vi "Controller Board Thermal Test.vi"(9 "Line In Voltage":dbl format="%#_13g", 10 "Power Supply In":string, 11 "DMM In":string) -> (3 "Temperature":dbl)   [LabVIEW 2013]
doc: "After applying maximum voltage and maximum ambient temperature, measure the temperature of the controller board."
uses:
  <instrlib>/Driver Simulation/DMM/TemperatureSensorTypes.ctl
  <instrlib>/Driver Simulation/Fixture.lvlib
  <instrlib>/Driver Simulation/Power Supply.lvlib
  <instrlib>/Driver Simulation/DMM.lvlib
panel:
  out "error out":errorcluster
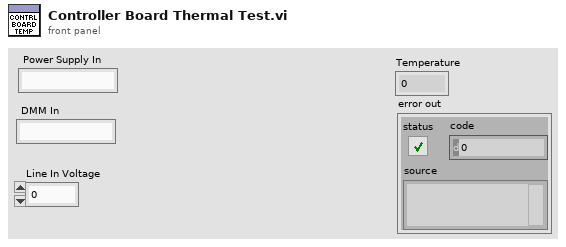
[diagram p1: front panel]
types:
  T1 = typedef "Driver Simulation.lvlib/DMM.lvlib/TemperatureSensorTypes.ctl" = i32
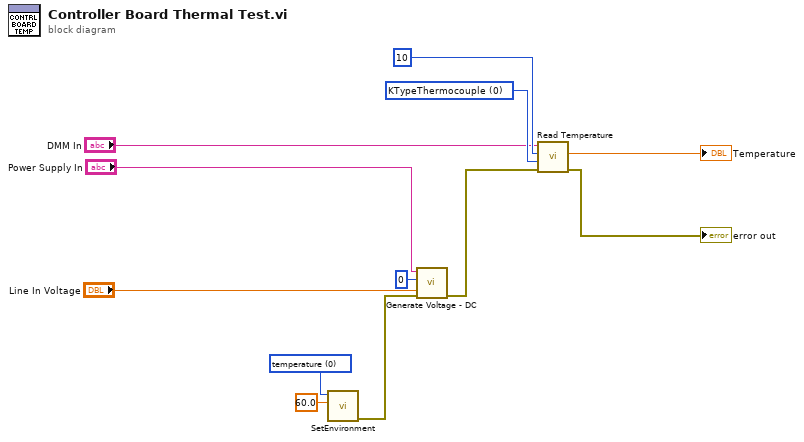
[diagram p0: block diagram]
diagram:
  w4 = T1 0 items=["KTypeThermocouple", "JTypeThermocouple"] ("sensorType")
  w12 = 0 items=["temperature", "light"] ("setting")
  n1 = call <instrlib>:"SetEnvironment.vi"("Value"=60.0 ("value"), "Setting"=w12) -> ("error out"=w8:errorcluster)  [unwired: 9 in]
  n2 = call <instrlib>:"Generate Voltage - DC.vi"("error in (no error)"=w8, "Output Voltage"="Line In Voltage", "Channel"=0 ("channel"), "Power Supply in"="Power Supply In") -> ("error out"=w2:errorcluster)  [unwired: 6 in, 1 out]
  n3 = call <instrlib>:"Read Temperature.vi"("error in (no error)"=w2, "Sensor Type"=w4, "Channel"=10 ("DMM Channel"), "DMM in"="DMM In") -> ("error out"=→"error out":errorcluster, "Temperature (C)"=→"Temperature":dbl)  [unwired: 5 in, 1 out]
